vi "Gamepad Controls to Robot Commands.vi"(11 "Robot Controls":T2) -> (3 "Robot Commands":T1)   [LabVIEW 2014]
uses:
  Robot Control Outputs 2015.ctl
  Robot Commands.ctl
  Global Variables/Miscalleneous.vi
  Global Variables/Settings.vi
panel:
  # "Field Centric"
  # "CB = control board"
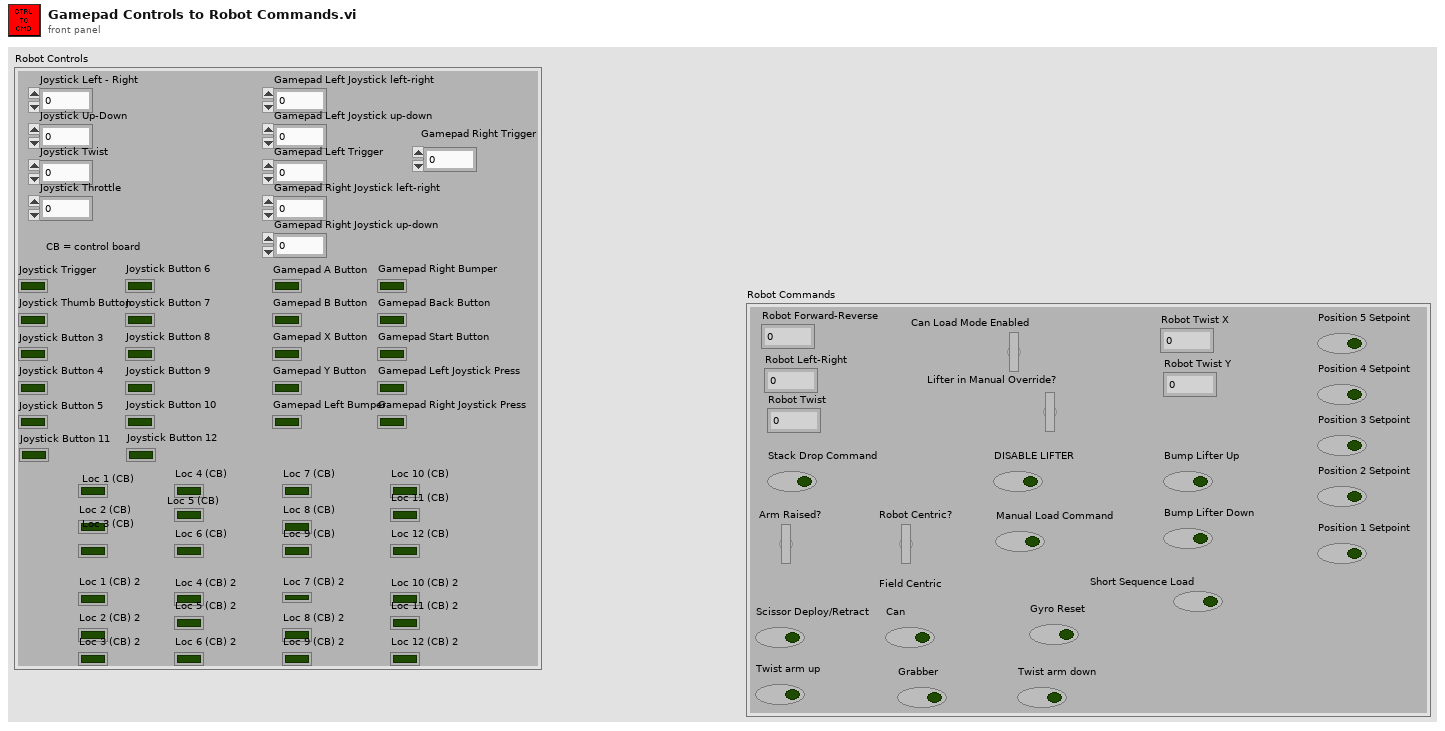
[diagram p1: front panel]
types:
  T1 = typedef "Robot Commands.ctl" = cluster{"Robot Forward-Reverse":dbl, "Robot Left-Right":dbl, "Robot Twist":dbl, "Can Load Mode Enabled":bool, "Lifter in Manual Override?":bool, "Stack Drop Command":bool, "Arm Raised?":bool, "DISABLE LIFTER":bool, "Position 1 Setpoint":bool, "Position 2 Setpoint":bool, "Position 3 Setpoint":bool, "Position 4 Setpoint":bool, "Position 5 Setpoint":bool, "Bump Lifter Down":bool, "Bump Lifter Up":bool, "Manual Load Command":bool, "Robot Centric?":bool, "Scissor Deploy/Retract":bool, "Grabber":bool, "Can":bool, "Twist arm up":bool, "Gyro Reset":bool, "Twist arm down":bool, "Short Sequence Load":bool, "Robot Twist X":dbl, "Robot Twist Y":dbl}
  T2 = typedef "Robot Control Outputs 2015.ctl" = cluster{"Gamepad Left Joystick left-right":dbl, "Gamepad Left Joystick up-down":dbl, "Gamepad A Button":bool, "Gamepad B Button":bool, "Gamepad X Button":bool, "Gamepad Y Button":bool, "Gamepad Left Bumper":bool, "Gamepad Right Bumper":bool, "Gamepad Back Button":bool, "Gamepad Start Button":bool, "Gamepad Left Joystick Press":bool, "Gamepad Right Joystick Press":bool, "Joystick Trigger":bool, "Joystick Thumb Button":bool, "Joystick Button 3":bool, "Joystick Button 4":bool, "Joystick Button 5":bool, "Joystick Button 6":bool, "Joystick Button 7":bool, "Joystick Button 8":bool, "Joystick Button 9":bool, "Joystick Button 10":bool, "Gamepad Left Trigger":dbl, "Gamepad Right Joystick left-right":dbl, "Gamepad Right Joystick up-down":dbl, "Joystick Left - Right":dbl, "Joystick Up-Down":dbl, "Joystick Twist":dbl, "Joystick Throttle":dbl, "Loc 1 (CB)":bool, "Loc 4 (CB)":bool, "Gamepad Right Trigger":dbl, "Loc 2 (CB)":bool, "Loc 3 (CB)":bool, "Loc 5 (CB)":bool, "Loc 6 (CB)":bool, "Loc 7 (CB)":bool, "Loc 10 (CB)":bool, "Loc 8 (CB)":bool, "Loc 9 (CB)":bool, "Loc 11 (CB)":bool, "Loc 12 (CB)":bool, "Joystick Button 11":bool, "Joystick Button 12":bool, "Loc 1 (CB) 2":bool, "Loc 4 (CB) 2":bool, "Loc 2 (CB) 2":bool, "Loc 3 (CB) 2":bool, "Loc 5 (CB) 2":bool, "Loc 6 (CB) 2":bool, "Loc 7 (CB) 2":bool, "Loc 10 (CB) 2":bool, "Loc 8 (CB) 2":bool, "Loc 9 (CB) 2":bool, "Loc 11 (CB) 2":bool, "Loc 12 (CB) 2":bool}
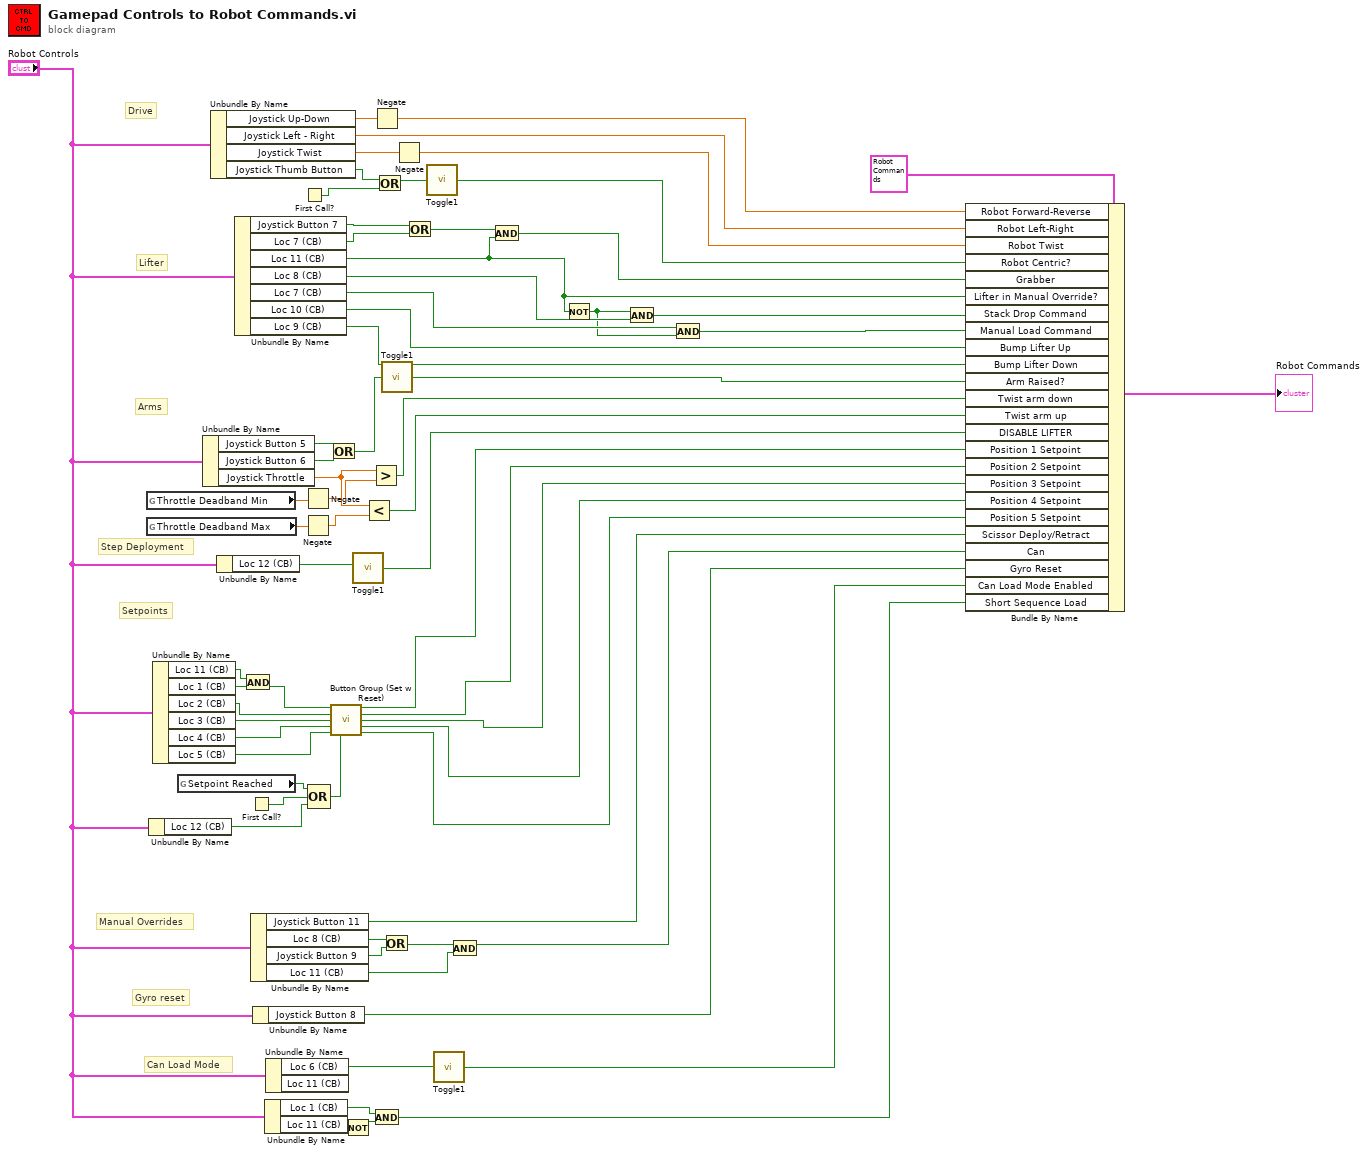
[diagram p0: block diagram]
diagram:
  # "Can Load Mode"
  # "Gyro reset"
  # "Manual Overrides"
  # "Setpoints"
  # "Step Deployment"
  # "Arms"
  # "Drive"
  # "Lifter"
  n1 = global read "Settings.vi" "Throttle Deadband Min"() -> (w45:dbl)
  n2 = global read "Settings.vi" "Throttle Deadband Max"() -> (w44:dbl)
  n3 = Unbundle By Name("Robot Controls") -> ("Loc 12 (CB)"=w53:bool)
  n4 = Unbundle By Name("Robot Controls") -> ("Loc 11 (CB)"=w17:bool, "Loc 1 (CB)"=w19:bool, "Loc 2 (CB)"=w28:bool, "Loc 3 (CB)"=w29:bool, "Loc 4 (CB)"=w30:bool, "Loc 5 (CB)"=w31:bool)
  n5 = global read "Miscalleneous.vi" "Setpoint Reached"() -> (w56:bool)
  n6 = Unbundle By Name("Robot Controls") -> ("Joystick Button 5"=w50:bool, "Joystick Button 6"=w51:bool, "Joystick Throttle"=w46:dbl)
  n7 = Unbundle By Name("Robot Controls") -> ("Joystick Up-Down"=w64:dbl, "Joystick Left - Right"=w63:dbl, "Joystick Twist"=w62:dbl, "Joystick Thumb Button"=w27:bool)
  n8 = Unbundle By Name("Robot Controls") -> ("Loc 12 (CB)"=w52:bool)
  n9 = Unbundle By Name("Robot Controls") -> ("Joystick Button 7"=w40:bool, "Loc 7 (CB)"=w39:bool, "Loc 11 (CB)"=w7:bool, "Loc 8 (CB)"=w2:bool, "Loc 7 (CB)"=w5:bool, "Loc 10 (CB)"=w61:bool, "Loc 9 (CB)"=w23:bool)
  n10 = And(x=w17, y=w19) -> (x .and. y?=w18:bool)
  n11 = First Call?() -> (First Call?: T/F=w57:bool)
  n12 = Unbundle By Name("Robot Controls") -> ("Joystick Button 11"=w54:bool, "Loc 8 (CB)"=w55:bool, "Joystick Button 9"=w20:bool, "Loc 11 (CB)"=w8:bool)
  n13 = Unbundle By Name("Robot Controls") -> ("Joystick Button 8"=w41:bool)
  n14 = Unbundle By Name("Robot Controls") -> ("Loc 1 (CB)"=w13:bool, "Loc 11 (CB)"=w14:bool)
  n15 = Unbundle By Name("Robot Controls") -> ("Loc 6 (CB)"=w3:bool)  [unwired: 1 out]
  n16 = First Call?() -> (First Call?: T/F=w25:bool)
  n17 = Negate(x=w45) -> (-x=w42:dbl)
  n18 = Negate(x=w44) -> (-x=w43:dbl)
  n19 = Compound Arithmetic op=OR(w56, w57, w53) -> (w32:bool)
  n20 = Or(x=w50, y=w51) -> (x .or. y?=w49:bool)
  n21 = call "Button Group (Set w Reset).vi"("Button 1"=w18, "Button 2"=w28, "Button 3"=w29, "Button 4"=w30, "Button 5"=w31, "Universal Reset"=w32) -> ("Button 1 out"=w37:bool, "Button 2 out"=w36:bool, "Button 3 out"=w35:bool, "Button 4 out"=w34:bool, "Button 5 out"=w33:bool)  [unwired: 5 in]
  n22 = Not(x=w14) -> (.not. x?=w12:bool)
  n23 = call "Toggle1.vi"("Boolean"=w52) -> ("Driver Switch 2"=w22:bool)
  n24 = Less?(x=w46, y=w43) -> (x < y?=w47:bool)
  n25 = Greater?(x=w46, y=w42) -> (0:w48:bool)
  n26 = Negate(x=w64) -> (-x=w60:dbl)
  n27 = And(x=w13, y=w12) -> (x .and. y?=w11:bool)
  n28 = Or(x=w27, y=w25) -> (x .or. y?=w26:bool)
  n29 = call "Toggle1.vi"("Boolean"=w49) -> ("Driver Switch 2"=w16:bool)
  n30 = Or(x=w55, y=w20) -> (x .or. y?=w21:bool)
  n31 = Negate(x=w62) -> (-x=w59:dbl)
  n32 = Or(x=w40, y=w39) -> (x .or. y?=w38:bool)
  n33 = call "Toggle1.vi"("Boolean"=w26) -> ("Driver Switch 2"=w58:bool)
  n34 = call "Toggle1.vi"("Boolean"=w3) -> ("Driver Switch 2"=w24:bool)
  n35 = And(x=w21, y=w8) -> (x .and. y?=w9:bool)
  n36 = And(x=w38, y=w7) -> (x .and. y?=w10:bool)
  n37 = Not(x=w7) -> (.not. x?=w1:bool)
  n38 = And(x=w1, y=w2) -> (x .and. y?=w4:bool)
  n39 = And(x=w5, y=w1) -> (x .and. y?=w6:bool)
  n40 = Bundle By Name(cluster=T1 {"Robot Forward-Reverse"=0.0, "Robot Left-Right"=0.0, "Robot Twist"=0.0, "Can Load Mode Enabled"=FALSE, "Lifter in Manual Override?"=FALSE, "Stack Drop Command"=FALSE, "Arm Raised?"=FALSE, "DISABLE LIFTER"=FALSE, "Position 1 Setpoint"=FALSE, "Position 2 Setpoint"=FALSE, "Position 3 Setpoint"=FALSE, "Position 4 Setpoint"=FALSE, "Position 5 Setpoint"=FALSE, "Bump Lifter Down"=FALSE, "Bump Lifter Up"=FALSE, "Manual Load Command"=FALSE, "Robot Centric?"=FALSE, "Scissor Deploy/Retract"=FALSE, "Grabber"=FALSE, "Can"=FALSE, "Twist arm up"=FALSE, "Gyro Reset"=FALSE, "Twist arm down"=FALSE, "Short Sequence Load"=FALSE, "Robot Twist X"=0.0, "Robot Twist Y"=0.0} ("Robot Controls 2"), "Robot Forward-Reverse"=w60, "Robot Left-Right"=w63, "Robot Twist"=w59, "Robot Centric?"=w58, "Grabber"=w10, "Lifter in Manual Override?"=w7, "Stack Drop Command"=w4, "Manual Load Command"=w6, "Bump Lifter Up"=w61, "Bump Lifter Down"=w23, "Arm Raised?"=w16, "Twist arm down"=w48, "Twist arm up"=w47, "DISABLE LIFTER"=w22, "Position 1 Setpoint"=w37, "Position 2 Setpoint"=w36, "Position 3 Setpoint"=w35, "Position 4 Setpoint"=w34, "Position 5 Setpoint"=w33, "Scissor Deploy/Retract"=w54, "Can"=w9, "Gyro Reset"=w41, "Can Load Mode Enabled"=w24, "Short Sequence Load"=w11) -> (→"Robot Commands":T1)
